vi "Prime BSI Camera Messenger.vi"(0 "Notifier Name":string, 2 "Prime Actions":T5, 5 "Prime Parameter":T2, 7 "ROI Setup":T1, 9 "# of Frames":u32, 11 "File Save Path":path) -> (4 "Notifier Name (Dup)":string, 6 "Prime Parameter":T2, 8 "Prime ROI":T1, 10 "Running?":bool, 13 "Image Ref":T4, 15 "Error?":bool)   [LabVIEW 2016]
uses:
  Prime BSI Controls/Prime Actions.ctl
  Prime BSI Controls/Prime Parameters.ctl
  Prime BSI Controls/Prime Parameter List.ctl
  Prime BSI Controls/Prime ROI.ctl
  <vilib>/vision/Image Controls.llb/IMAQ Image.ctl
  Prime BSI Controls/Prime Notifier Element.ctl
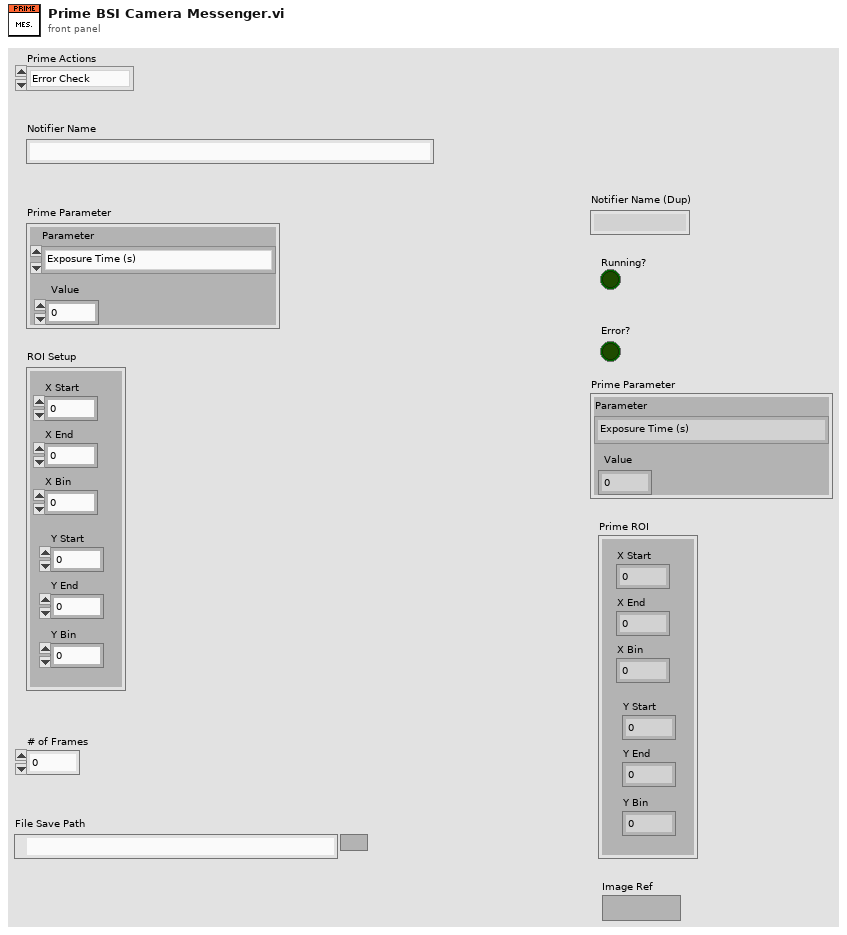
[diagram p1: front panel]
types:
  T1 = typedef "Prime ROI.ctl" = cluster{"X Start":u32, "X End":u32, "X Bin":u32, "Y Start":u32, "Y End":u32, "Y Bin":u32}
  T2 = typedef "Prime Parameters.ctl" = cluster{"Parameter":T3, "Value":dbl}
  T3 = typedef "Prime Parameter List.ctl" = enum16{"Exposure Time (s)"}
  T4 = typedef "IMAQ Image.ctl" = refnum<image>
  T5 = typedef "Prime Actions.ctl" = enum16{"Error Check", "Initialize", "Preview", "Record", "Abort", "Record Settings", "Set Parameter", "Get Parameter", "Set ROI", "Get ROI", "Status", "Set Trigger", "Quit"}
  T6 = typedef "Prime Notifier Element.ctl" = cluster{"Prime Actions":T5, "Received?":bool, "Prime Parameter":T2, "Prime ROI":T1, "Running?":bool, "File Path":path, "# of frames":u32, "Image Ref":T4, "Error":errorcluster}
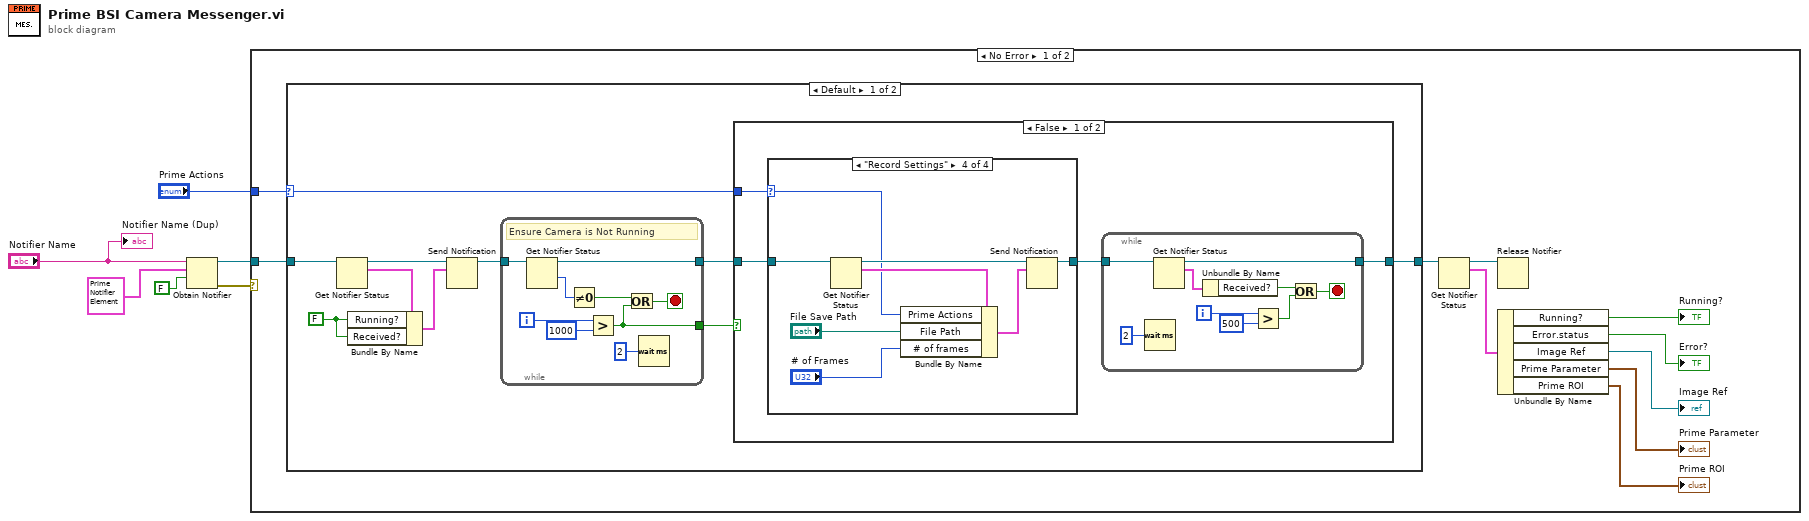
[diagram p0: block diagram]
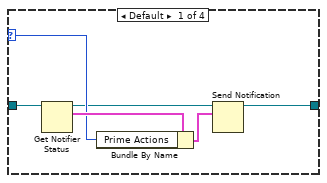
[diagram p2: hidden frame]
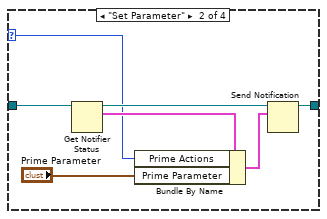
[diagram p3: hidden frame]
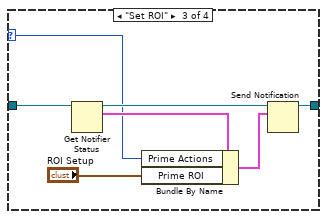
[diagram p4: hidden frame]
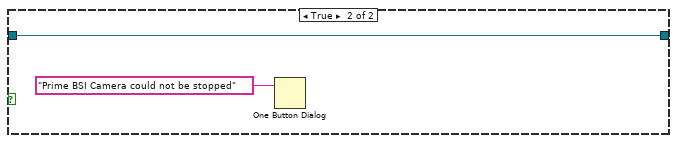
[diagram p5: hidden frame]
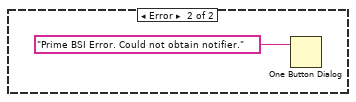
[diagram p7: hidden frame]
diagram:
  n1 = Obtain Notifier(name (unnamed)="Notifier Name", notification data type=T6 {"Prime Actions"=enum."Error Check", "Received?"=FALSE, "Prime Parameter"={"Parameter"=enum."Exposure Time (s)", "Value"=0.0}, "Prime ROI"={"X Start"=0, "X End"=0, "X Bin"=0, "Y Start"=0, "Y End"=0, "Y Bin"=0}, "Running?"=FALSE, "File Path"=path "", "# of frames"=0, "Image Ref"=refnum, "Error"={"status"=FALSE, "code"=0, "source"=""}} ("Prime Camera Cluster"), create if not found? (T)=FALSE) -> (notifier out=w4:refnum<notifier>, error out=w5:errorcluster)  [unwired: 1 in, 1 out]
  n2 = case shown="No Error" w5 {
    tunnel: w4 -> [w16 _]
    tunnel: "Prime Actions" -> [w15 _]
    frame No Error {
      n3 = case shown="Default" w15 {
        selector: w15 -> [w22 _]
        tunnel: w16 -> [w26 w79]
        tunnel: [w21 w79] -> w14
        frame Default {
          w17 = FALSE ("Running?")
          n4 = Get Notifier Status(notifier=w26) -> (notifier out=w20:refnum<notifier>, current notification=w19:T6)  [unwired: 1 in, 3 out]
          n5 = Bundle By Name(cluster=w19, "Running?"=w17, "Received?"=w17) -> (w18:T6)
          n6 = Send Notification(notification=w18, notifier=w20) -> (notifier out=w25:refnum<notifier>)  [unwired: 1 in, 1 out]
          n7 = while {
            tunnel: w25 -> [w78]
            tunnel: [w77] -> w23
            tunnel: [w72] -> w24
            i -> [w74]
            stop <- w76 stop-if-true
            # "Ensure Camera is Not Running"
            n8 = Get Notifier Status(notifier=w78) -> (notifier out=w77:refnum<notifier>, # waiting=w71:i32)  [unwired: 1 in, 3 out]
            n9 = Not Equal To 0?(x=w71) -> (x != 0?=w70:bool)
            n10 = Greater?(x=w74, y=1000) -> (0:w72:bool)
            n11 = Or(x=w70, y=w72) -> (x .or. y?=w76:bool)
            n12 = Wait (ms)(milliseconds to wait=u32 2) -> ()  [unwired: 1 out]
          }
          n13 = case shown="False" w24 {
            tunnel: w23 -> [w28 w68]
            tunnel: w22 -> [w30 _]
            tunnel: [w27 w68] -> w21
            frame False {
              n14 = case shown="\"Record Settings\"" w30 {
                selector: w30 -> [w43 w47 w54 w62]
                tunnel: w28 -> [w45 w52 w59 w67]
                tunnel: [w40 w50 w57 w65] -> w29
                frame Default {
                  n15 = Get Notifier Status(notifier=w45) -> (notifier out=w42:refnum<notifier>, current notification=w44:T6)  [unwired: 1 in, 3 out]
                  n16 = Bundle By Name(cluster=w44, "Prime Actions"=w43) -> (w41:T6)
                  n17 = Send Notification(notification=w41, notifier=w42) -> (notifier out=w40:refnum<notifier>)  [unwired: 1 in, 1 out]
                }
                frame "Set Parameter" {
                  n18 = Get Notifier Status(notifier=w52) -> (notifier out=w51:refnum<notifier>, current notification=w49:T6)  [unwired: 1 in, 3 out]
                  n19 = Bundle By Name(cluster=w49, "Prime Actions"=w47, "Prime Parameter"="Prime Parameter") -> (w48:T6)
                  n20 = Send Notification(notification=w48, notifier=w51) -> (notifier out=w50:refnum<notifier>)  [unwired: 1 in, 1 out]
                }
                frame "Set ROI" {
                  n21 = Get Notifier Status(notifier=w59) -> (notifier out=w58:refnum<notifier>, current notification=w56:T6)  [unwired: 1 in, 3 out]
                  n22 = Bundle By Name(cluster=w56, "Prime Actions"=w54, "Prime ROI"="ROI Setup") -> (w55:T6)
                  n23 = Send Notification(notification=w55, notifier=w58) -> (notifier out=w57:refnum<notifier>)  [unwired: 1 in, 1 out]
                }
                frame "Record Settings" {
                  n24 = Get Notifier Status(notifier=w67) -> (notifier out=w66:refnum<notifier>, current notification=w64:T6)  [unwired: 1 in, 3 out]
                  n25 = Bundle By Name(cluster=w64, "Prime Actions"=w62, "File Path"="File Save Path", "# of frames"="# of Frames") -> (w63:T6)
                  n26 = Send Notification(notification=w63, notifier=w66) -> (notifier out=w65:refnum<notifier>)  [unwired: 1 in, 1 out]
                }
              }
              n27 = while {
                tunnel: w29 -> [w39]
                tunnel: [w31] -> w27
                i -> [w36]
                stop <- w32 stop-if-true
                n28 = Wait (ms)(milliseconds to wait=u32 2) -> ()  [unwired: 1 out]
                n29 = Get Notifier Status(notifier=w39) -> (notifier out=w31:refnum<notifier>, current notification=w38:T6)  [unwired: 1 in, 3 out]
                n30 = Unbundle By Name(w38) -> ("Received?"=w37:bool)
                n31 = Greater?(x=w36, y=500) -> (0:w34:bool)
                n32 = Or(x=w37, y=w34) -> (x .or. y?=w32:bool)
              }
            }
            frame True {
              n33 = One Button Dialog(message="Prime BSI Camera could not be stopped") -> ()  [unwired: 1 in, 1 out]
            }
          }
        }
        frame "Status" {
        }
      }
      n34 = Get Notifier Status(notifier=w14) -> (notifier out=w13:refnum<notifier>, current notification=w12:T6)  [unwired: 1 in, 3 out]
      n35 = Release Notifier(notifier=w13) -> ()  [unwired: 2 in, 3 out]
      n36 = Unbundle By Name(w12) -> ("Running?"=→"Running?":bool, "Error.status"=→"Error?":bool, "Image Ref"=→"Image Ref":T4, "Prime Parameter"=→"Prime Parameter":T2, "Prime ROI"=→"Prime ROI":T1)
    }
    frame Error {
      n37 = One Button Dialog(message="Prime BSI Error. Could not obtain notifier.") -> ()  [unwired: 1 in, 1 out]
    }
  }
  "Notifier Name (Dup)" <- "Notifier Name"
